vi "Push Button.vi"(8 "error in (no error)":errorcluster, 10 "Button":T1, 11 "Inst.FP in":refnum<class "Inst.FP.lvclass">) -> (0 "error out":errorcluster, 3 "Inst.FP out":refnum<class "Inst.FP.lvclass">)   [LabVIEW 2019, in "Inst.FP.lvclass"]
uses:
  Inst.FP.lvclass
  C:/Program Files (x86)/National Instruments/LabVIEW 2019/user.lib/LevyLab/Instrument Framework/SMOs/Instrument/Instrument.lvclass
  Typedefs/Inst.FP.Buttons--Enum.ctl
  Typedefs/Inst.FP.Commands--Enum.ctl
  Typedefs/Inst.FP.Push Button--Cluster.ctl
  <userlib>/LevyLab/Instrument Framework/SMOs/Instrument/Instrument.lvclass/Instrument.ctl
  67792bfe-8e2c-4879-abc2-cb448bcec168.vi
  67792bfe-8e2c-4879-abc2-cb448bcec168.vi/e6734212-7c9e-4ce8-a442-683b18d6b7e6.vi
  <userlib>/LevyLab/Instrument Framework/SMOs/Instrument/API/Send and Receive.vi
  67792bfe-8e2c-4879-abc2-cb448bcec168.vi/d08038f8-4acd-46a3-976f-e1cbe8915b66.vi
  <userlib>/LevyLab/Instrument Framework/SMOs/Instrument/Private/Get Client Type.vi
  67792bfe-8e2c-4879-abc2-cb448bcec168.vi/e6734212-7c9e-4ce8-a442-683b18d6b7e6.vi/4333ab82-ae47-474b-91ed-9005e4c3f9aa.vi
  67792bfe-8e2c-4879-abc2-cb448bcec168.vi/e6734212-7c9e-4ce8-a442-683b18d6b7e6.vi/d37b70f9-b0d2-43c7-93ce-5cddff78440f.vi
  67792bfe-8e2c-4879-abc2-cb448bcec168.vi/d08038f8-4acd-46a3-976f-e1cbe8915b66.vi/800cf9c4-7383-40cf-9bc6-eb11c7b09f2f.vi
  67792bfe-8e2c-4879-abc2-cb448bcec168.vi/d08038f8-4acd-46a3-976f-e1cbe8915b66.vi/0f5049b1-9107-4d80-b470-81422f3edf74.vi
  67792bfe-8e2c-4879-abc2-cb448bcec168.vi/d08038f8-4acd-46a3-976f-e1cbe8915b66.vi/800cf9c4-7383-40cf-9bc6-eb11c7b09f2f.vi/24dfb1b4-dc66-422d-bf6c-4b679291b096.vi
  67792bfe-8e2c-4879-abc2-cb448bcec168.vi/d08038f8-4acd-46a3-976f-e1cbe8915b66.vi/800cf9c4-7383-40cf-9bc6-eb11c7b09f2f.vi/89a5d855-98d7-49e5-b538-c332b2d9e0ac.vi
  <userlib>/LevyLab/Instrument Framework/SMOs/Instrument/Private/Get RC Connection Status.vi
  <userlib>/LevyLab/Instrument Framework/SMOs/Instrument/API/Enum to String.vi
  <userlib>/LevyLab/Instrument Framework/SMOs/RemoteControl/API/Send and Receive.vi
  <vilib>/Utility/Data Type/Get Type Information.vi
  <vilib>/JDP Science/JSONtext/JSON text to Variant.vi
  <userlib>/LevyLab/Instrument Framework/SMOs/Instrument/API/Instrument.GetPublicEvents.vi
  <vilib>/JDP Science/JSONtext/Variant to JSON Text.vi
  <vilib>/National Instruments/GUID Generator/Guid Generator.vi
  <userlib>/LevyLab/Instrument Framework/SMOs/Instrument/API/Instrument.MessageToProcess.vi
  <userlib>/LevyLab/Instrument Framework/SMOs/Instrument/Private/Instrument.MessageFromProcess.EventStructure.vi
  <vilib>/JDP Science/JSONtext/LVClass Serializer/JSONtext LVClass Serializer.lvclass
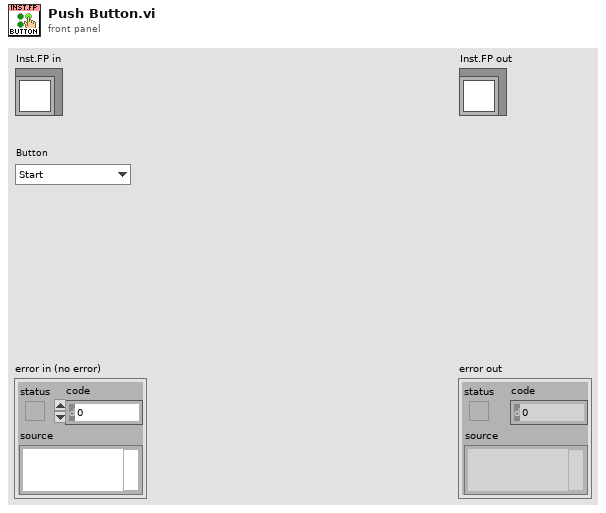
[diagram p1: front panel]
types:
  T1 = typedef "Inst.FP.lvclass/Inst.FP.Buttons--Enum.ctl" = enum16{"Start", "3He", "4He", "Normal", "Recovery", "Auto", "LED Test", "Reset"}
  T2 = typedef "Inst.FP.lvclass/Inst.FP.Push Button--Cluster.ctl" = cluster{"Button":T1}
  T3 = typedef "Inst.FP.lvclass/Inst.FP.Commands--Enum.ctl" = enum16{"Get Mode", "Set Mode", "Push Button"}
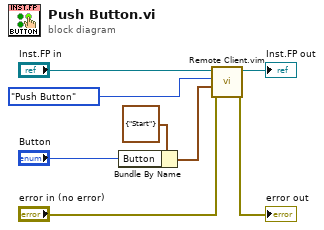
[diagram p0: block diagram]
diagram:
  n1 = Bundle By Name(cluster=T2 {"Button"=enum."Start"} ("Push Button"), "Button"="Button") -> (w2:T2)
  n2 = call "Remote Client.vim"("error in (no error)"="error in (no error)", "params"=w2, "method"=Inst.FP.Commands--Enum."Push Button" ("Commands"), "Instrument in"="Inst.FP in") -> ("error out"=→"error out":errorcluster, "Instrument out"=→"Inst.FP out":refnum<class "Inst.FP.lvclass">)  [unwired: 4 in, 2 out]
